vi "Auton move distance.vi"(0 "Distance":dbl=3.0 format="%#_13g", 1 "PID gains":T1={"proportional gain (Kc)"=1.0, "integral time (Ti, min)"=0.01, "derivative time (Td, min)"=0.0} {"derivative time (Td, min)" format="%.3f"; "integral time (Ti, min)" format="%.3f"; "proportional gain (Kc)" format="%.3f"}, 3 "Refnum in":refnum<k33>) -> (7 "Distance Travelled":dbl)   [LabVIEW 2014]
uses:
  Lightning base/TeleopCmd.ctl
  Lightning base/CmdFlag.ctl
  <vilib>/addons/control/pid/pid.llb/PID (DBL).vi
  <vilib>/addons/control/pid/NI_PID_pid.lvlib
panel:
  in  "output cluster 2":T1
  out "dt out (s)":dbl format="%.3f"
  out "PID output":dbl format="%.2f"
  out "Boolean 2":bool
  out "Boolean":bool
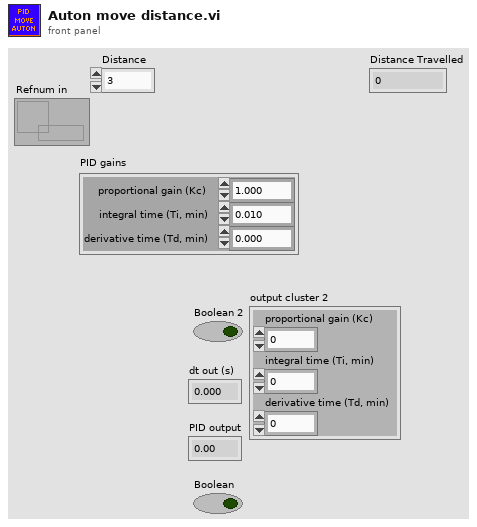
[diagram p1: front panel]
types:
  T1 = cluster{"proportional gain (Kc)":dbl, "integral time (Ti, min)":dbl, "derivative time (Td, min)":dbl}
  T2 = typedef "TeleopCmd.ctl" = cluster{"Left Joystick":dbl, "Right Joystick":dbl, "Shift":bool, "CmdFlag":T3}
  T3 = typedef "CmdFlag.ctl" = enum16{"noop", "suspend", "resume"}
  T4 = typedef "WPI_EncoderDevRef.ctl" = cluster{"DevStatus":errorcluster, "EncoderIndex":T5, "CounterIndex":T6, "DistancePerCount":dbl, "Decoding Type":T7}
  T5 = typedef "FPGA_EncoderIdx.ctl" = enum8{"Enc 0", "Enc 1", "Enc 2", "Enc 3", "Enc 4", "Enc 5", "Enc 6", "Enc 7", "Invalid"}
  T6 = typedef "FPGA_CounterCtrSystemIndex.ctl" = enum8{"Ctr 0", "Ctr 1", "Ctr 2", "Ctr 3", "Ctr 4", "Ctr 5", "Ctr 6", "Ctr 7", "Invalid"}
  T7 = typedef "WPI_EncoderType.ctl" = enum16{"1x", "2x", "4x"}
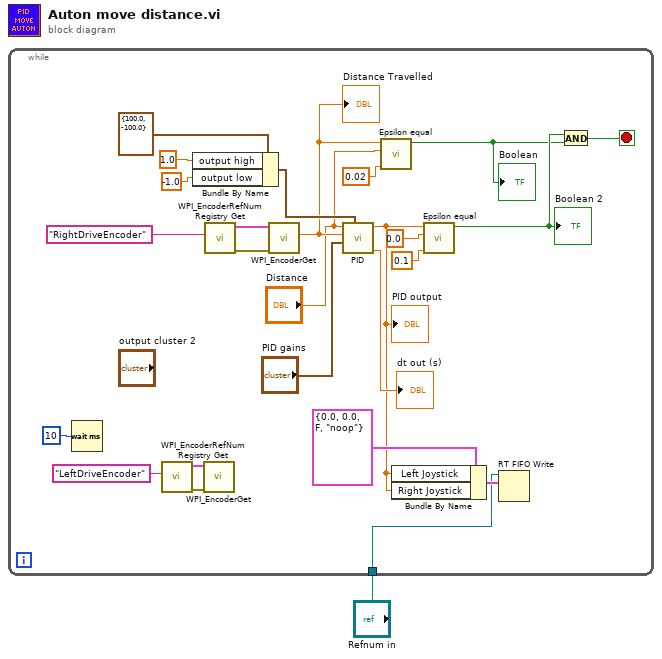
[diagram p0: block diagram]
diagram:
  n1 = while {
    tunnel: "Refnum in" -> [w4]
    stop <- w14 stop-if-true
    n2 = Wait (ms)(milliseconds to wait=u32 10) -> ()  [unwired: 1 out]
    n3 = call <vilib>:"WPI_EncoderRefNum Registry Get.vi"("refnum name"="LeftDriveEncoder") -> ("error out"=w22:errorcluster, "EncoderDevRef"=w23:T4)  [unwired: 9 in]
    n4 = Bundle By Name(cluster=cluster{"output high":dbl, "output low":dbl} {"output high"=100.0, "output low"=-100.0} ("output range"), "output high"=1.0, "output low"=-1.0) -> (w19:cluster{"output high":dbl, "output low":dbl})
    n5 = call <vilib>:"WPI_EncoderGet.vi"("error in (no error)"=w22, "EncoderDevRef"=w23) -> ()  [unwired: 4 in, 6 out]
    n6 = call <vilib>:"WPI_EncoderRefNum Registry Get.vi"("refnum name"="RightDriveEncoder") -> ("error out"=w25:errorcluster, "EncoderDevRef"=w26:T4)  [unwired: 9 in]
    n7 = call <vilib>:"WPI_EncoderGet.vi"("error in (no error)"=w25, "EncoderDevRef"=w26) -> ("Distance"=w8:dbl)  [unwired: 4 in, 5 out]
    "Distance Travelled" <- w8
    n8 = call-poly <vilib>:"PID.vi"("output range"=w19, "PID gains"="PID gains", "process variable"=w8, "setpoint"="Distance") -> ("dt out (s)"=→"dt out (s)":dbl, "output"=w6:dbl)  [unwired: 6 in]
    "PID output" <- w6
    n9 = call "Epsilon equal.vi"("Epsilon"=0.02, "Value2"="Distance", "Value1"=w8) -> ("Boolean"=w12:bool)  [unwired: 8 in]
    "Boolean" <- w12
    n10 = Bundle By Name(cluster=T2 {"Left Joystick"=0.0, "Right Joystick"=0.0, "Shift"=FALSE, "CmdFlag"=enum."noop"} ("Cluster"), "Left Joystick"=w6, "Right Joystick"=w6) -> (w5:T2)
    n11 = call "Epsilon equal.vi"("Epsilon"=0.1, "Value2"=0.0, "Value1"=w6) -> ("Boolean"=w13:bool)  [unwired: 8 in]
    "Boolean 2" <- w13
    n12 = RT FIFO Write(0:w4, 1:w5) -> ()  [unwired: 3 in, 4 out]
    n13 = And(x=w13, y=w12) -> (x .and. y?=w14:bool)
  }
